vi "GT Get Capture Offset Status.vi"(0 "cardNum":i16, 1 "pCapturePos":i32, 5 "encoder":i16, 7 "pCount":i16, 9 "pLoop":i32, 11 "error in (no error)":errorcluster caption="错误输入（无错误）") -> (3 "pCapturePos out":i32, 4 "function return":i16, 8 "pCount out":i16, 10 "pLoop out":i32, 15 "error out":errorcluster caption="错误输出")   [LabVIEW 2020, in "gts1.lvlib"]
doc: "GT_API GT_GetCaptureOffsetStatus(short cardNum,short encoder,short *pCount,long *pLoop,long *pCapturePos);"
uses:
  gts1.lvlib
  dll/32bit/multi_card/gts.dll
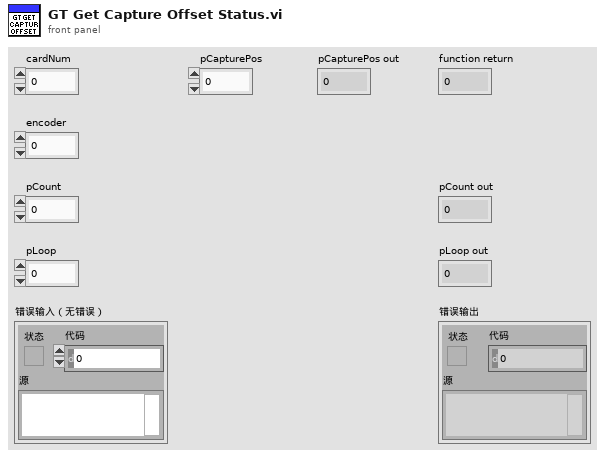
[diagram p1: front panel]
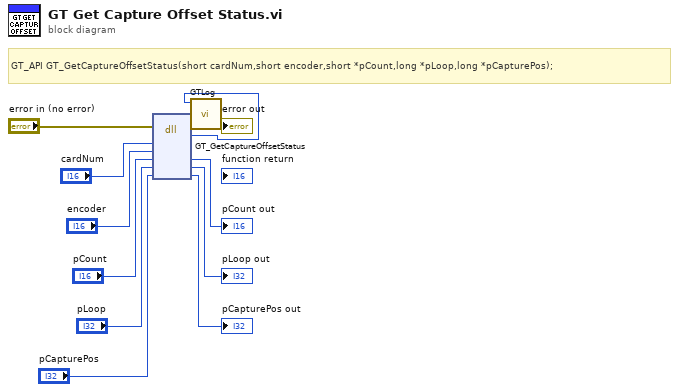
[diagram p0: block diagram]
diagram:
  # "GT_API GT_GetCaptureOffsetStatus(short cardNum,short encoder,short *pCount,long *pLoop,long *pCapturePos);"
  n1 = dll-call lib="C:/1228/dll/32bit/multi_card/gts.dll" fn="GT_GetCaptureOffsetStatus"(error in="error in (no error)", "cardNum"="cardNum", "encoder"="encoder", "pCount"="pCount", "pLoop"="pLoop", "pCapturePos"="pCapturePos") -> (error out=w3:errorcluster, w1:i16, "pCount"=→"pCount out":i16, "pLoop"=→"pLoop out":i32, "pCapturePos"=→"pCapturePos out":i32)  [unwired: 4 in, 1 out]
  n2 = call "GTLog.vi"("error in (no error)"=w3, "Numeric"=w1) -> ("error out"=→"error out":errorcluster)  [unwired: 9 in]
